vi "PictureRotation_171213.vi"(8 "Cluster":cluster{i16, i32, i16, i32}, 9 "FullTrack":bool, 10 "Segments":bool, 11 "Angle":dbl) -> (3 "Array":u32[][](array[numeric]))   [LabVIEW 2016]
uses:
  Globaltracker.vi
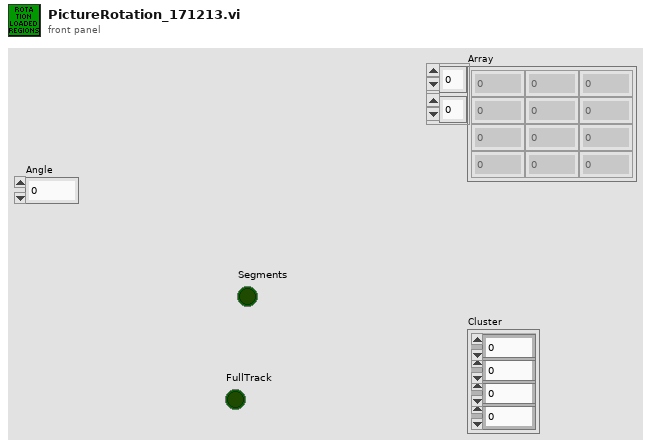
[diagram p1: front panel]
types:
  T1 = typedef "imagedata.ctl" = cluster{"image type":i32, "image depth":i32, "image":u8[], "mask":u8[], "colors":u32[], "Rectangle":cluster{"left":i16, "top":i16, "right":i16, "bottom":i16}}
  T2 = cluster{"left":i16, "top":i16, "right":i16, "bottom":i16}
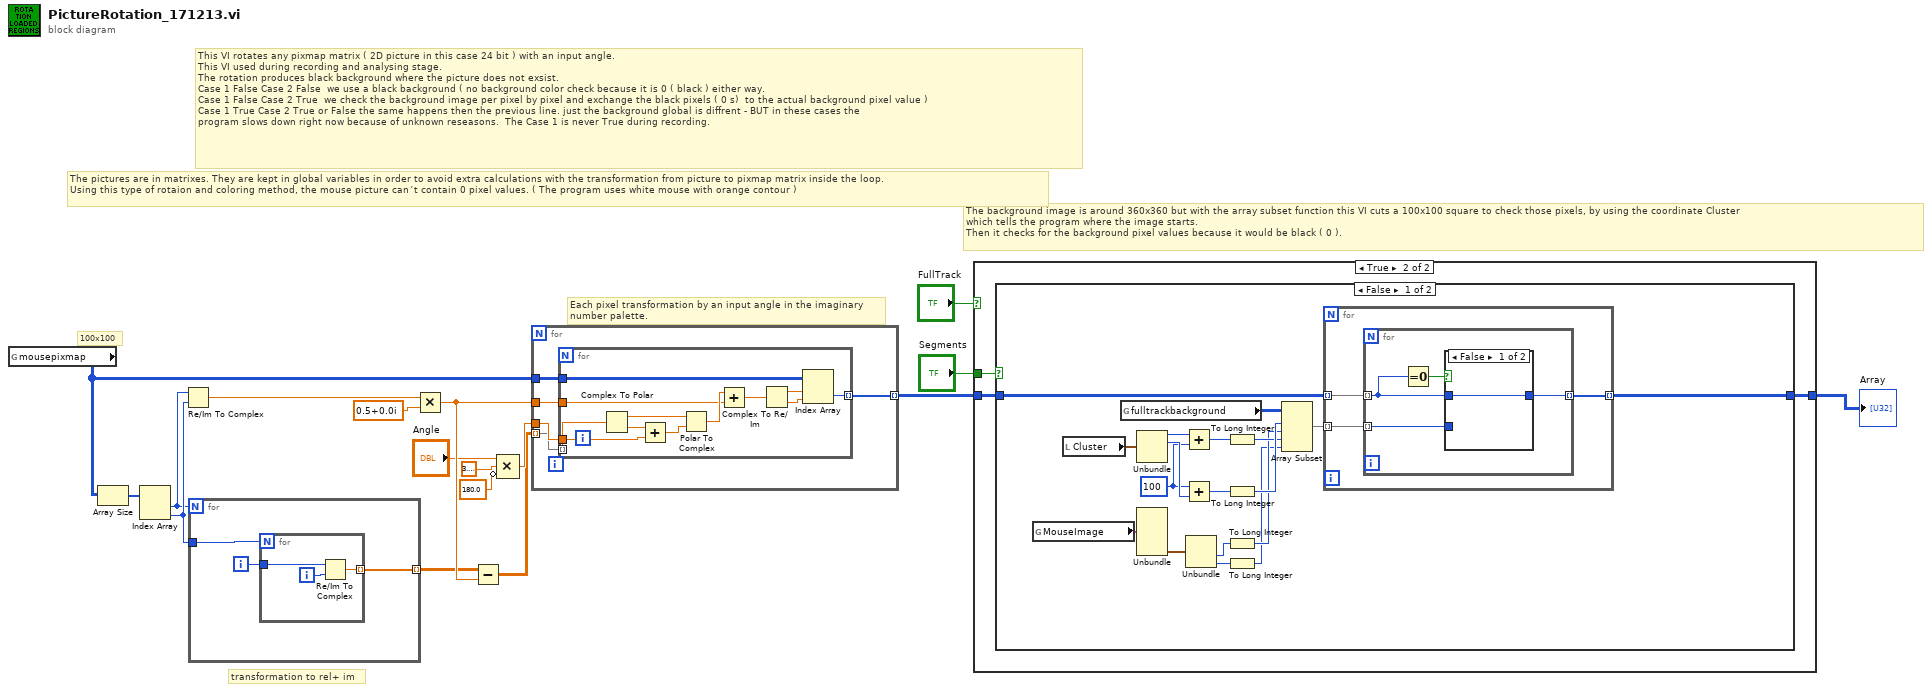
[diagram p0: block diagram]
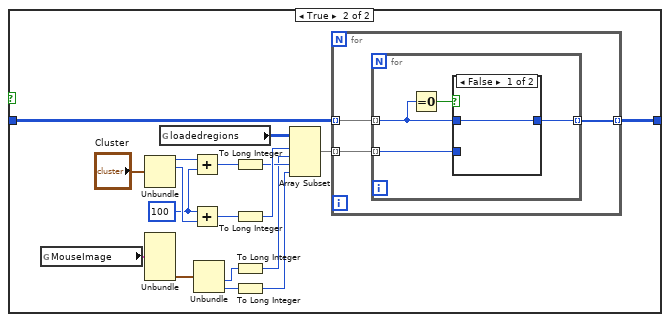
[diagram p3: hidden frame]
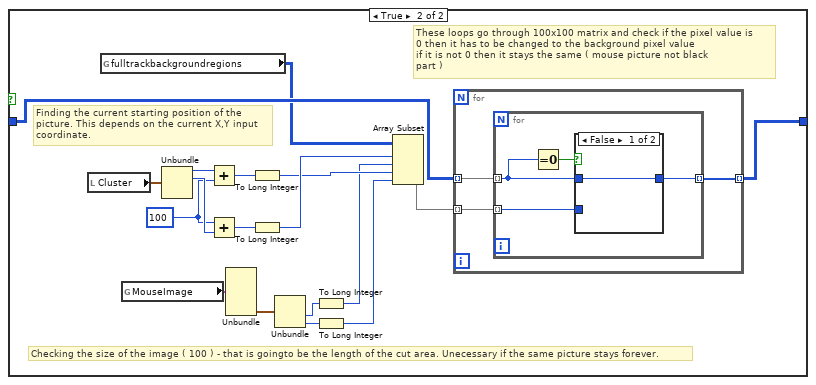
[diagram p6: hidden frame]
diagram:
  # "The background image is around 360x360 but with the array subset function this VI cuts a 100x100 square to check those pixels, by using the coordinate Cluster \nwhich tells the program where the image starts. \nThen it checks for the background pixel values because it would be black ( 0 )."
  # "Each pixel transformation by an input angle in the imaginary \nnumber palette."
  # "transformation to rel+ im"
  # "100x100"
  # "The pictures are in matrixes. They are kept in global variables in order to avoid extra calculations with the transformation from picture to pixmap matrix inside the loop.\nUsing this type of rotaion and coloring method, the mouse picture can´t contain 0 pixel values. ( The program uses white mouse with orange contour )"
  # "This VI rotates any pixmap matrix ( 2D picture in this case 24 bit ) with an input angle.\nThis VI used during recording and analysing stage.\nThe rotation produces black background where the picture does not exsist.\nCase 1 False Case 2 False  we use a black background ( no background color check because it is 0 ( black ) either way. \nCase 1 False Case 2 True  we check the background image per pixel by pixel and exchange the black pixels ( 0 s)  to the actual background pixel value )\nCase 1 True Case 2 True or False the same happens then the previous line. just the background global is diffrent - BUT in these cases the \nprogram slows down right now because of unknown reseasons.  The Case 1 is never True during recording."
  n1 = global read "Globaltracker.vi" "mousepixmap"() -> (w3:u32[][])
  n2 = Array Size(array=w3) -> (size(s)=w17:i32[])
  n3 = Index Array(array=w17) -> (element #1=w7:i32, element #2=w8:i32)  [unwired: 2 in]
  n4 = Re/Im To Complex(1:w8, 2:w7) -> (0:w11:cdb)
  n5 = for {
    N: w7 -> [_]
    tunnel: [w19] -> w6 mode=indexing
    tunnel: w8 -> [w18]
    i -> [w20]
    n6 = for {
      N: w18 -> [_]
      tunnel: w20 -> [w22]
      tunnel: [w21] -> w19 mode=indexing
      i -> [w23]
      n7 = Re/Im To Complex(1:w23, 2:w22) -> (0:w21:cdb)
    }
  }
  n8 = Multiply(x=w11, y=cdb 0.5+0.0i) -> (x*y=w12:cdb)
  n9 = Subtract(x=w6, y=w12) -> (x-y=w10:cdb[][])
  n10 = Compound Arithmetic op=MULTIPLY("Angle", 3.141592653589793, invert 180.0 ("value")) -> (w15:dbl)
  n11 = for {
    tunnel: w15 -> [w28]
    tunnel: w3 -> [w27]
    tunnel: w12 -> [w26]
    tunnel: w10 -> [w25] mode=indexing
    tunnel: [w24] -> w5 mode=indexing
    n12 = for {
      tunnel: w27 -> [w34]
      tunnel: w28 -> [w37]
      tunnel: w26 -> [w31]
      tunnel: w25 -> [w30] mode=indexing
      tunnel: [w29] -> w24 mode=indexing
      n13 = Complex To Polar(r * e^(i*theta)=w30) -> (r=w40:dbl, theta=w39:dbl)
      n14 = Add(x=w39, y=w37) -> (x+y=w38:dbl)
      n15 = Polar To Complex(1:w38, 2:w40) -> (0:w36:cdb)
      n16 = Add(x=w36, y=w31) -> (x+y=w32:cdb)
      n17 = Complex To Re/Im(x + iy=w32) -> (x=w35:dbl, y=w33:dbl)
      n18 = Index Array(array=w34, index (row)=w35, index (col)=w33) -> (element=w29:u32)
    }
  }
  n19 = case shown="True" "FullTrack" {
    tunnel: w5 -> [w43 w74]
    tunnel: [w42 w73] -> w4
    tunnel: "Segments" -> [w41 w72]
    frame False {
      n20 = case shown="False" w41 {
        tunnel: w43 -> [w44 w62]
        tunnel: [w44 w60] -> w42
        frame False {
        }
        frame True {
          w46 = i16 100 ("y")
          n21 = global read "Globaltracker.vi" "MouseImage"() -> (w56:T1)
          n22 = Unbundle("Cluster") -> (w50:i16, w49:i32)  [unwired: 2 out]
          n23 = Unbundle(w56) -> ("Rectangle"=w55:T2)  [unwired: 5 out]
          n24 = global read "Globaltracker.vi" "loadedregions"() -> (w57:u32[][])
          n25 = Add(x=w50, y=w46) -> (x+y=w48:i16)
          n26 = Add(x=w46, y=w49) -> (x+y=w47:i32)
          n27 = Unbundle(w55) -> ("right"=w54:i16, "bottom"=w53:i16)  [unwired: 2 out]
          n28 = To Long Integer(number=w48) -> (32bit integer=w58:i32)
          n29 = To Long Integer(number=w47) -> (32bit integer=w59:i32)
          n30 = To Long Integer(number=w54) -> (32bit integer=w52:i32)
          n31 = To Long Integer(number=w53) -> (32bit integer=w51:i32)
          n32 = Array Subset(array=w57, index (row)=w59, length (row)=w52, index (col)=w58, length (col)=w51) -> (w61:u32[][])
          n33 = for {
            tunnel: w62 -> [w65] mode=indexing
            tunnel: [w64] -> w60 mode=indexing
            tunnel: w61 -> [w63] mode=indexing
            n34 = for {
              tunnel: w65 -> [w67] mode=indexing
              tunnel: [w68] -> w64 mode=indexing
              tunnel: w63 -> [w66] mode=indexing
              n35 = Equal To 0?(x=w67) -> (x = 0?=w69:bool)
              n36 = case shown="False" w69 {
                tunnel: [w70 w71] -> w68
                tunnel: w67 -> [w70 _]
                tunnel: w66 -> [_ w71]
                frame False {
                }
                frame True {
                }
              }
            }
          }
        }
      }
    }
    frame True {
      n37 = case shown="False" w72 {
        tunnel: w74 -> [w76 w119]
        tunnel: [w75 w117] -> w73
        frame False {
          w77 = i16 100 ("y")
          n38 = global read "Globaltracker.vi" "MouseImage"() -> (w88:T1)
          n39 = local read "Cluster"() -> (w78:cluster{i16, i32, i16, i32})
          n40 = global read "Globaltracker.vi" "fulltrackbackground"() -> (w89:u32[][])
          n41 = Unbundle(w78) -> (w82:i16, w81:i32)  [unwired: 2 out]
          n42 = Unbundle(w88) -> ("Rectangle"=w87:T2)  [unwired: 5 out]
          n43 = Add(x=w82, y=w77) -> (x+y=w80:i16)
          n44 = Add(x=w77, y=w81) -> (x+y=w79:i32)
          n45 = Unbundle(w87) -> ("right"=w86:i16, "bottom"=w85:i16)  [unwired: 2 out]
          n46 = To Long Integer(number=w80) -> (32bit integer=w90:i32)
          n47 = To Long Integer(number=w79) -> (32bit integer=w91:i32)
          n48 = To Long Integer(number=w86) -> (32bit integer=w84:i32)
          n49 = To Long Integer(number=w85) -> (32bit integer=w83:i32)
          n50 = Array Subset(array=w89, index (row)=w91, length (row)=w84, index (col)=w90, length (col)=w83) -> (w92:u32[][])
          n51 = for {
            tunnel: w76 -> [w95] mode=indexing
            tunnel: [w94] -> w75 mode=indexing
            tunnel: w92 -> [w93] mode=indexing
            n52 = for {
              tunnel: w95 -> [w97] mode=indexing
              tunnel: [w98] -> w94 mode=indexing
              tunnel: w93 -> [w96] mode=indexing
              n53 = Equal To 0?(x=w97) -> (x = 0?=w99:bool)
              n54 = case shown="False" w99 {
                tunnel: [w100 w101] -> w98
                tunnel: w97 -> [w100 _]
                tunnel: w96 -> [_ w101]
                frame False {
                }
                frame True {
                }
              }
            }
          }
        }
        frame True {
          w103 = i16 100 ("y")
          # "These loops go through 100x100 matrix and check if the pixel value is \n0 then it has to be changed to the background pixel value\nif it is not 0 then it stays the same ( mouse picture not black \npart )"
          # "Finding the current starting position of the \npicture. This depends on the current X,Y input\ncoordinate."
          # "Checking the size of the image ( 100 ) - that is goingto be the length of the cut area. Unecessary if the same picture stays forever."
          n55 = local read "Cluster"() -> (w102:cluster{i16, i32, i16, i32})
          n56 = global read "Globaltracker.vi" "fulltrackbackgroundregions"() -> (w114:u32[][])
          n57 = global read "Globaltracker.vi" "MouseImage"() -> (w113:T1)
          n58 = Unbundle(w102) -> (w107:i16, w106:i32)  [unwired: 2 out]
          n59 = Add(x=w107, y=w103) -> (x+y=w105:i16)
          n60 = Add(x=w103, y=w106) -> (x+y=w104:i32)
          n61 = Unbundle(w113) -> ("Rectangle"=w112:T2)  [unwired: 5 out]
          n62 = To Long Integer(number=w105) -> (32bit integer=w115:i32)
          n63 = To Long Integer(number=w104) -> (32bit integer=w116:i32)
          n64 = Unbundle(w112) -> ("right"=w111:i16, "bottom"=w110:i16)  [unwired: 2 out]
          n65 = To Long Integer(number=w111) -> (32bit integer=w109:i32)
          n66 = To Long Integer(number=w110) -> (32bit integer=w108:i32)
          n67 = Array Subset(array=w114, index (row)=w116, length (row)=w109, index (col)=w115, length (col)=w108) -> (w118:u32[][])
          n68 = for {
            tunnel: w119 -> [w122] mode=indexing
            tunnel: [w121] -> w117 mode=indexing
            tunnel: w118 -> [w120] mode=indexing
            n69 = for {
              tunnel: w122 -> [w124] mode=indexing
              tunnel: [w125] -> w121 mode=indexing
              tunnel: w120 -> [w123] mode=indexing
              n70 = Equal To 0?(x=w124) -> (x = 0?=w126:bool)
              n71 = case shown="False" w126 {
                tunnel: [w127 w128] -> w125
                tunnel: w124 -> [w127 _]
                tunnel: w123 -> [_ w128]
                frame False {
                }
                frame True {
                }
              }
            }
          }
        }
      }
    }
  }
  "Array" <- w4
